vi "Example Stack Status.vi"() -> ()   [LabVIEW 2013]
uses:
  C:/tf/play/labview/Tinkerforge.dll
panel:
  out "stack current (A)":sgl
  out "stack voltage (V)":sgl
  in  "uid":string="6QjH3b"
  in  "port":i32=4223
  in  "host":string="localhost"
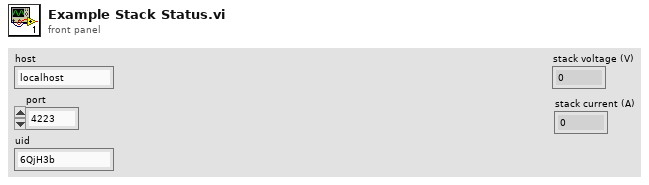
[diagram p1: front panel]
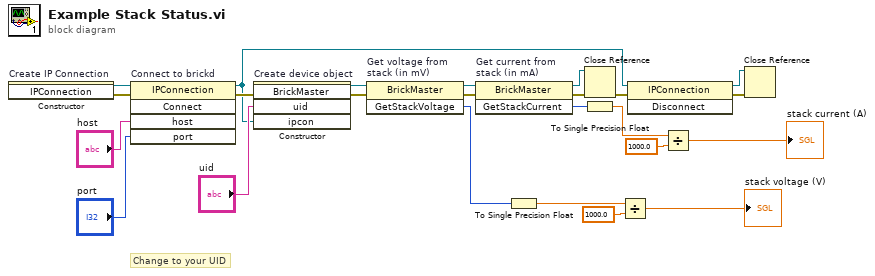
[diagram p0: block diagram]
diagram:
  # "Change to your UID"
  n1 = constructor on="Create IP Connection" class="IPConnection"() -> (reference out=w24:refnum<k24>, error out=w1:errorcluster)  [unwired: 3 in, 1 out]
  n2 = invoke on="Connect to brickd" class="IPConnection" method="Connect"(reference=w24, error in=w1, "host"="host", "port"="port") -> (reference out=w15:refnum<k24>, error out=w20:errorcluster)  [unwired: 1 in, 3 out]
  n3 = constructor on="Create device object" class="BrickMaster"(error in=w20, "uid"="uid", "ipcon"=w15) -> (reference out=w18:refnum<k24>, error out=w19:errorcluster)  [unwired: 2 in, 3 out]
  n4 = invoke on="Get voltage from\nstack (in mV)" class="BrickMaster" method="GetStackVoltage"(reference=w18, error in=w19) -> (reference out=w7:refnum<k24>, error out=w9:errorcluster, "GetStackVoltage"=w13:i32)  [unwired: 1 in]
  n5 = invoke on="Get current from\nstack (in mA)" class="BrickMaster" method="GetStackCurrent"(reference=w7, error in=w9) -> (reference out=w6:refnum<k24>, error out=w8:errorcluster, "GetStackCurrent"=w2:i32)  [unwired: 1 in]
  n6 = To Single Precision Float(number=w13) -> (single precision float=w11:sgl)
  n7 = Close Reference(reference=w6, error in (no error)=w8) -> (error out=w17:errorcluster)
  n8 = To Single Precision Float(number=w2) -> (single precision float=w4:sgl)
  n9 = Divide(x=w11, y=sgl 1000.0) -> (x/y=→"stack voltage (V)":sgl)
  n10 = invoke class="IPConnection" method="Disconnect"(reference=w15, error in=w17) -> (reference out=w14:refnum<k24>, error out=w16:errorcluster)  [unwired: 1 in, 1 out]
  n11 = Divide(x=w4, y=sgl 1000.0) -> (x/y=→"stack current (A)":sgl)
  n12 = Close Reference(reference=w14, error in (no error)=w16) -> ()  [unwired: 1 out]
